vi "Get BuildWorker Default Configuration.vi"(8 "error in (no error)":errorcluster, 11 "BuildWorker Controller in":refnum<class "BuildWorker Controller.lvclass">) -> (0 "error out":errorcluster, 2 "#Max Worker":i32, 3 "BuildWorker Controller out":refnum<class "BuildWorker Controller.lvclass">)   [LabVIEW 2017, in "BuildWorker Controller.lvlib" / "BuildWorker Controller.lvclass"]
uses:
  BuildWorker Controller.lvclass
  BuildWorker/BuildWorker.lvclass
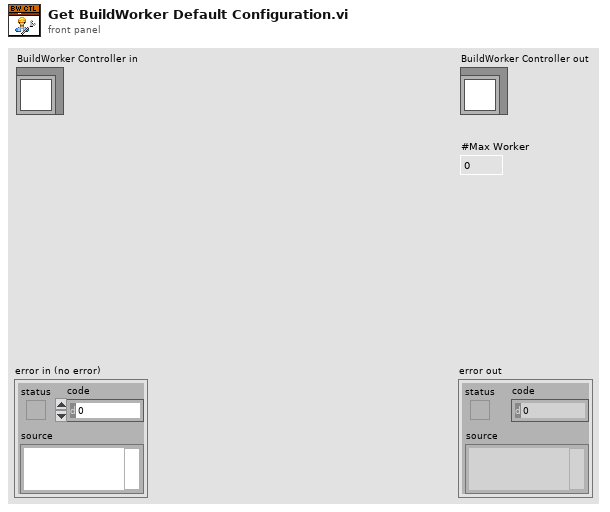
[diagram p1: front panel]
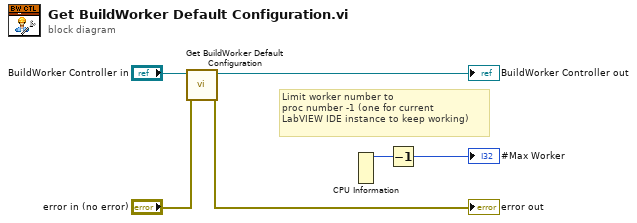
[diagram p0: block diagram]
diagram:
  # "Limit worker number to\nproc number -1 (one for current\nLabVIEW IDE instance to keep working)"
  n1 = call-parent "Get BuildWorker Default Configuration.vi"("error in (no error)"="error in (no error)", "BuildWorker in"="BuildWorker Controller in") -> ("error out"=→"error out":errorcluster, "BuildWorker out"=→"BuildWorker Controller out":refnum<class "BuildWorker Controller.lvclass">)  [unwired: 7 in, 1 out]
  n2 = CPU Information() -> (4:w5:i32)  [unwired: 3 out]
  n3 = Decrement(x=w5) -> (x-1=→"#Max Worker":i32)
